vi "DMD_start.vi"() -> (0 "error out":errorcluster, 3 "reference out":refnum<k24>)   [LabVIEW 2017]
panel:
  in  "FileName":string="C:\\Users\\1TEM\\Documents\\1TEM_control\\tem_image_loader\\bin\\Release\\tem_image_loader.exe"
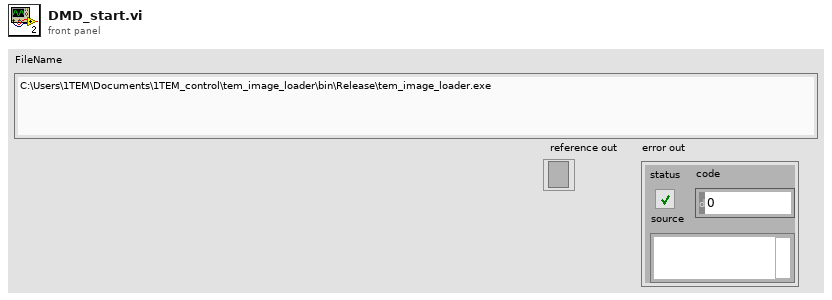
[diagram p1: front panel]
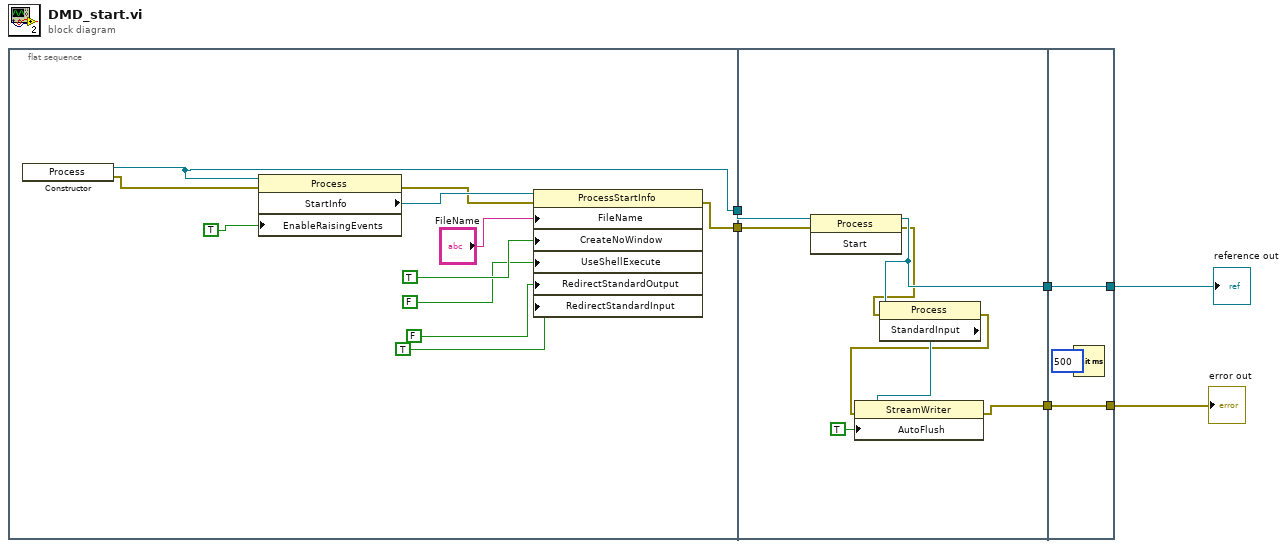
[diagram p0: block diagram]
diagram:
  n1 = flat-sequence {
    tunnel: [w11] -> w6
    tunnel: [w7] -> w4
    tunnel: w6 -> [w25]
    tunnel: w4 -> [w21]
    tunnel: [w22] -> w2
    tunnel: [w18] -> w1
    tunnel: [w27] -> w3
    tunnel: [w28] -> w5
    tunnel: w2 -> [w28]
    tunnel: w1 -> [w27]
    frame #0 {
      n2 = constructor class="Process"() -> (reference out=w11:refnum<k24>, error out=w9:errorcluster)  [unwired: 3 in, 1 out]
      n3 = property class="Process"(reference=w11, error in=w9, "EnableRaisingEvents"=TRUE) -> (error out=w8:errorcluster, "StartInfo"=w17:refnum<k24>)  [unwired: 1 out]
      n4 = property class="ProcessStartInfo"(reference=w17, error in=w8, "FileName"="FileName", "CreateNoWindow"=TRUE, "UseShellExecute"=FALSE, "RedirectStandardOutput"=FALSE, "RedirectStandardInput"=TRUE) -> (error out=w7:errorcluster)  [unwired: 1 out]
    }
    frame #1 {
      n5 = invoke class="Process" method="Start"(reference=w25, error in=w21) -> (reference out=w22:refnum<k24>, error out=w20:errorcluster)  [unwired: 1 in, 1 out]
      n6 = property class="Process"(reference=w22, error in=w20) -> (error out=w19:errorcluster, "StandardInput"=w24:refnum<k24>)  [unwired: 1 out]
      n7 = property class="StreamWriter"(reference=w24, error in=w19, "AutoFlush"=TRUE) -> (error out=w18:errorcluster)  [unwired: 1 out]
    }
    frame #2 {
      n8 = Wait (ms)(milliseconds to wait=u32 500) -> ()  [unwired: 1 out]
    }
  }
  "reference out" <- w5
  "error out" <- w3
